vi "srv_loop.vi"(8 "error in (no error)":errorcluster, 9 "Marker Queue":refnum<queue>, 10 "Server queue":refnum<queue>, 11 "Message Queues":T4) -> (0 "error out":errorcluster)   [LabVIEW 2013]
doc: "Message loop for handling messages pertaining to the acquisition of data from the hardware."
uses:
  queues/que_all_message_queues.ctl
  queues/que_message_cluster.ctl
  gui/type_def/general_and_device.ctl
  gui/type_def/general.ctl
  gui/type_def/device.ctl
  srv_state.ctl
  queues/que_enqueue_message_single.vi
  gui/global_var.vi
  <vilib>/Utility/error.llb/Error Cluster From Error Code.vi
  <vilib>/ErrorRing/Error Ring.xnode
panel:
  out "data_format":string
  out "fs":i32
  out "gral_&_device":T1={"general"={"file_ext"="0.0.0.0", "TCP port"=0, "#devices"=0, "log?"=FALSE, "tcp?"=FALSE, "language"="ENG"}, "eeg_device"={"name"="", "hardware"="", "image"="", "path"=path "", "extra"="", "channels"=""}}
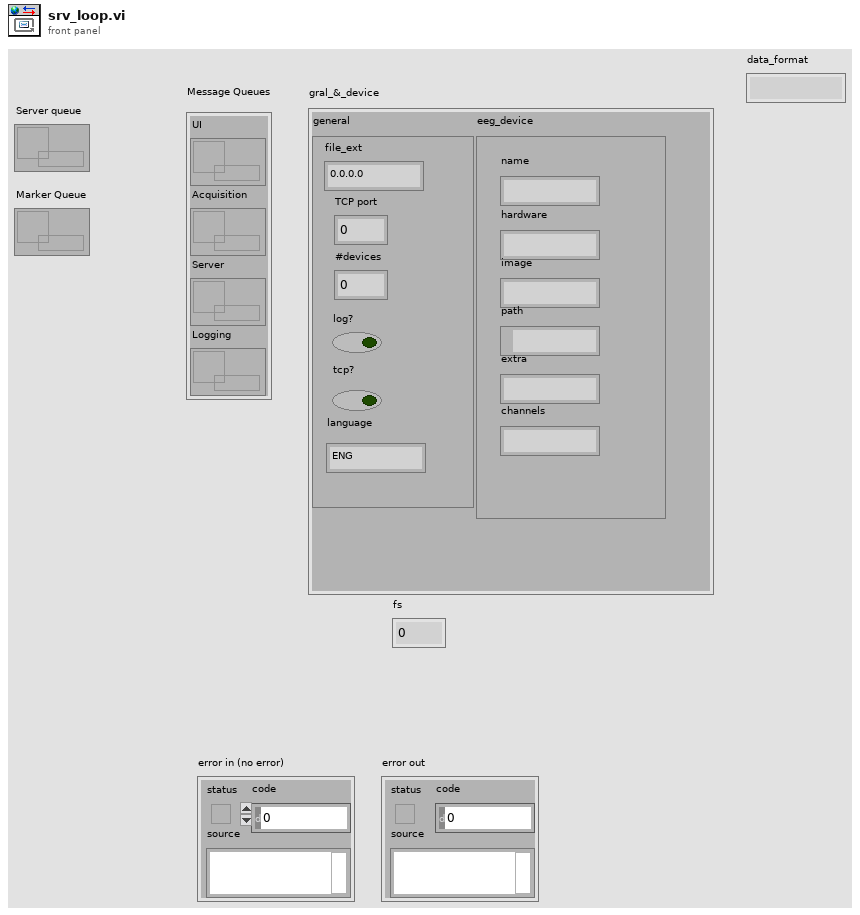
[diagram p1: front panel]
types:
  T1 = typedef "general_and_device.ctl" = cluster{"general":T2, "eeg_device":T3}
  T2 = typedef "general.ctl" = cluster{"file_ext":string, "TCP port":i32, "#devices":i32, "log?":bool, "tcp?":bool, "language":string}
  T3 = typedef "device.ctl" = cluster{"name":string, "hardware":string, "image":string, "path":path, "extra":string, "channels":string}
  T4 = typedef "que_all_message_queues.ctl" = cluster{"UI":refnum<queue>, "Acquisition":refnum<queue>, "Server":refnum<queue>, "Logging":refnum<queue>}
  T5 = typedef "srv_state.ctl" = enum16{"Idle", "Serving"}
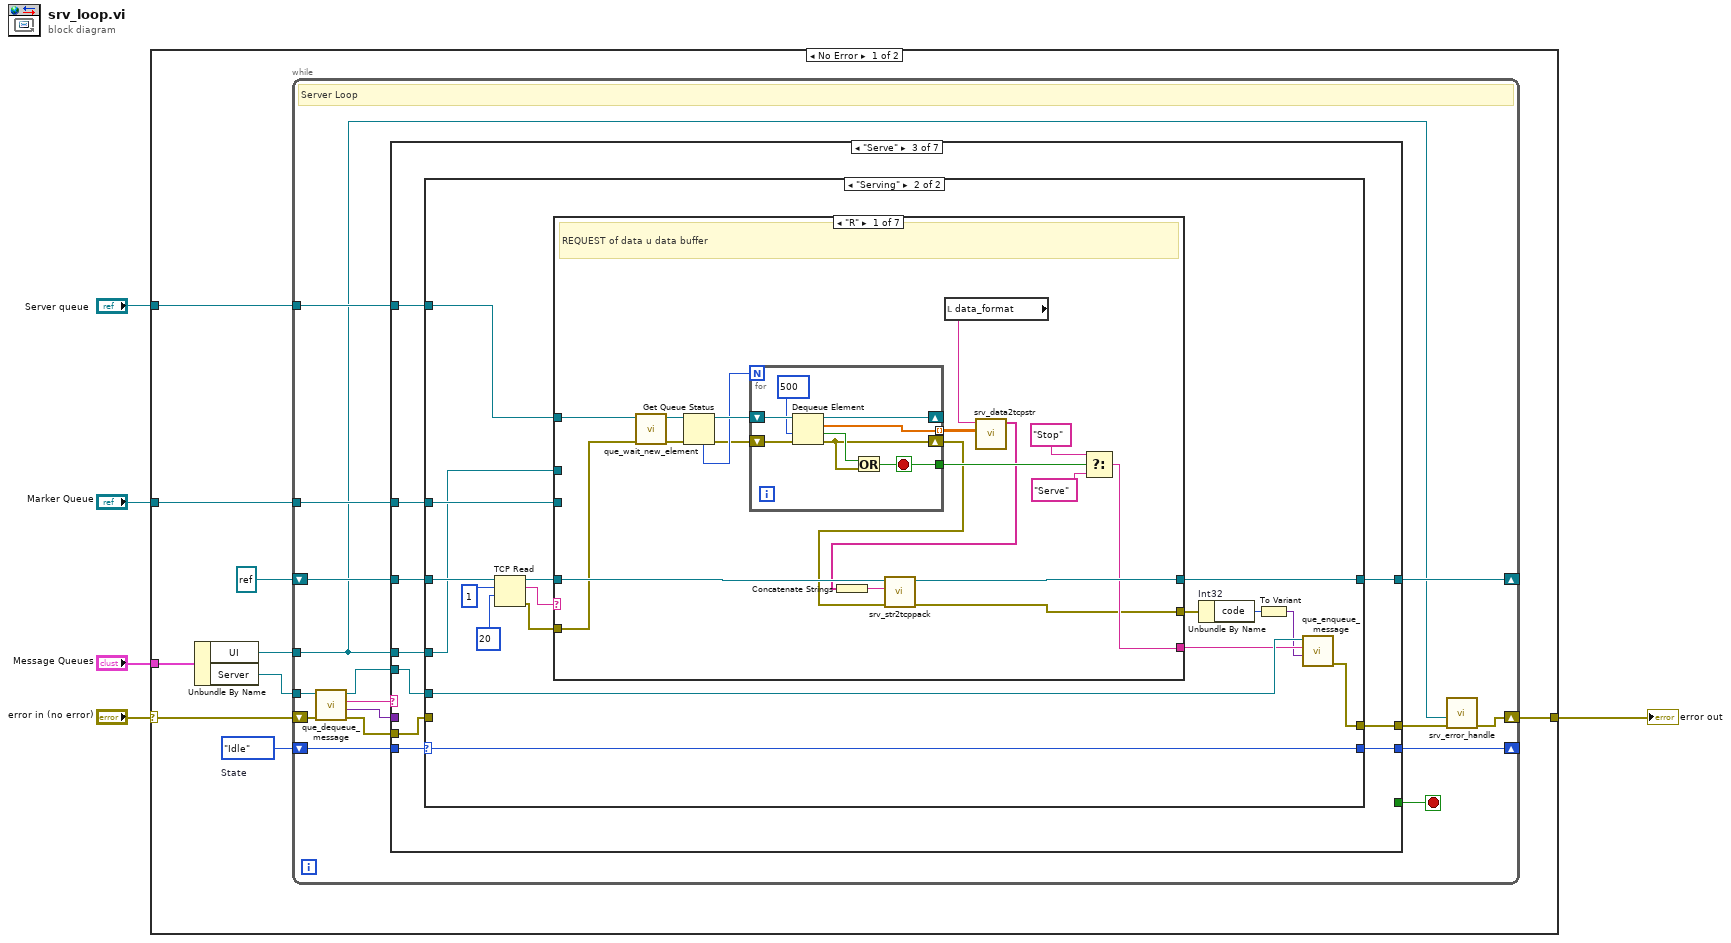
[diagram p0: block diagram]
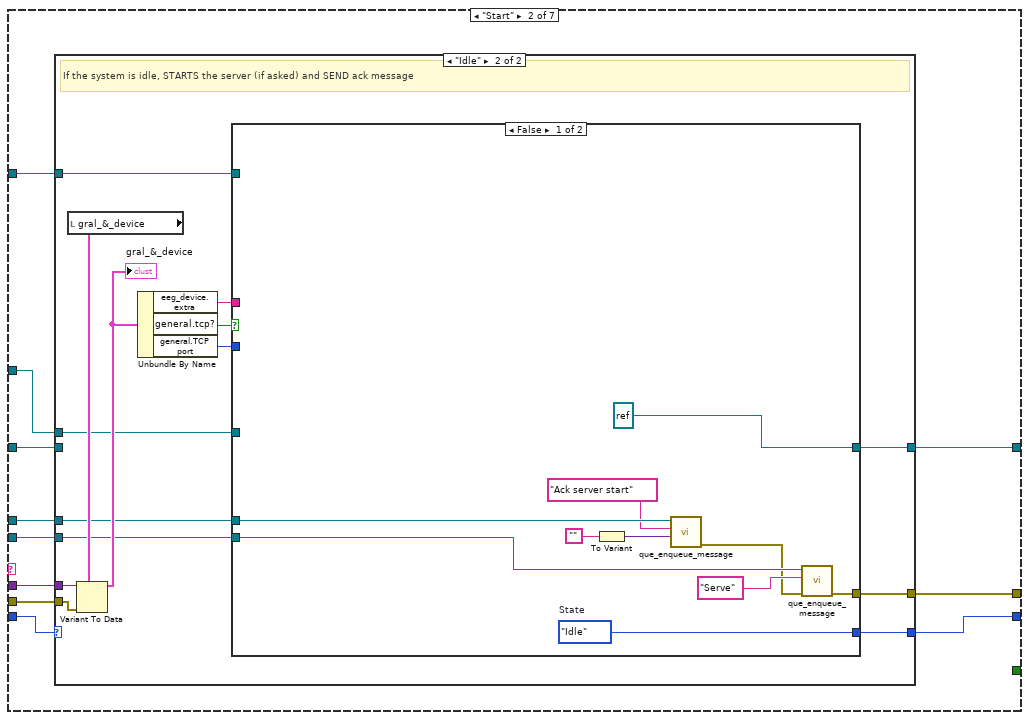
[diagram p3: hidden frame]
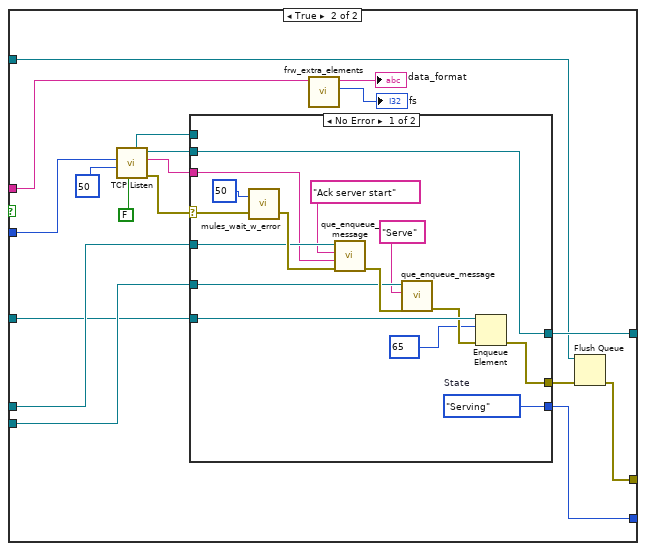
[diagram p5: hidden frame]
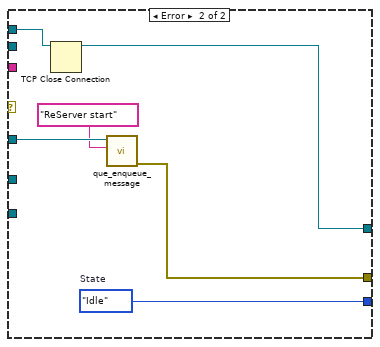
[diagram p6: hidden frame]
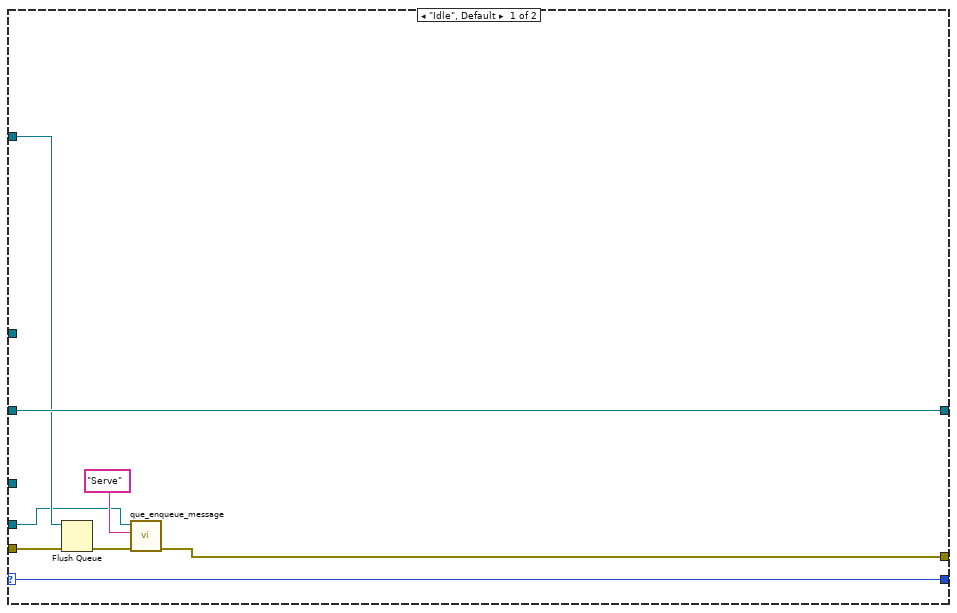
[diagram p7: hidden frame]
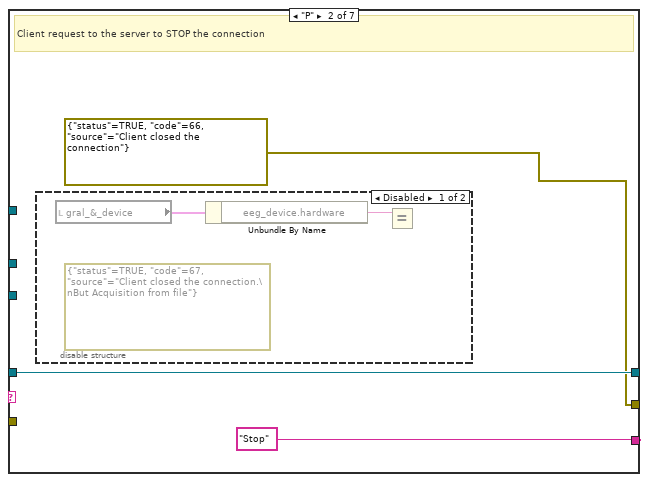
[diagram p8: hidden frame]
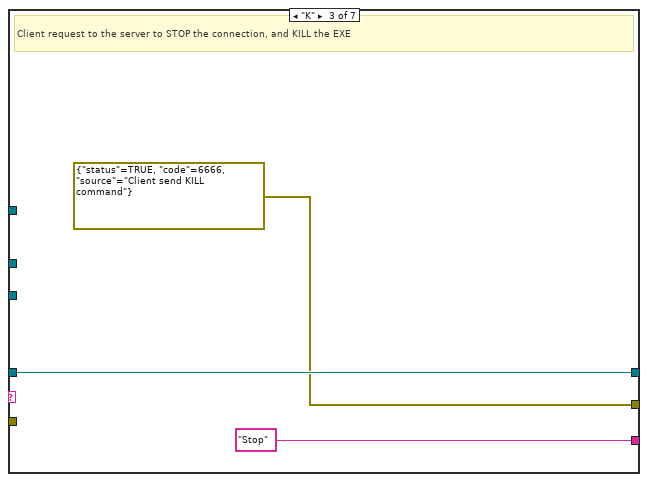
[diagram p10: hidden frame]
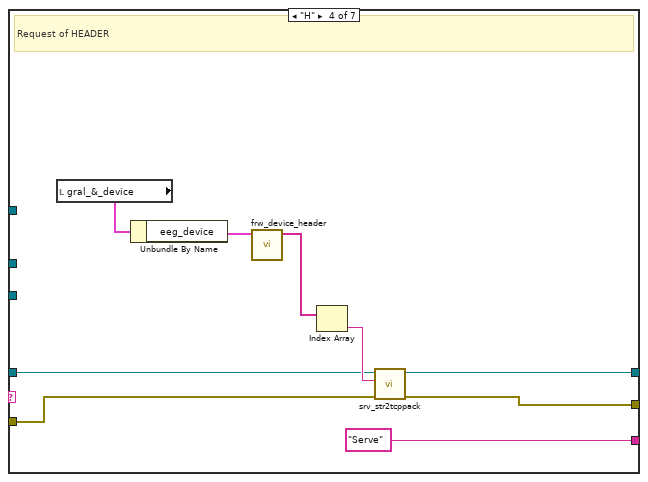
[diagram p11: hidden frame]
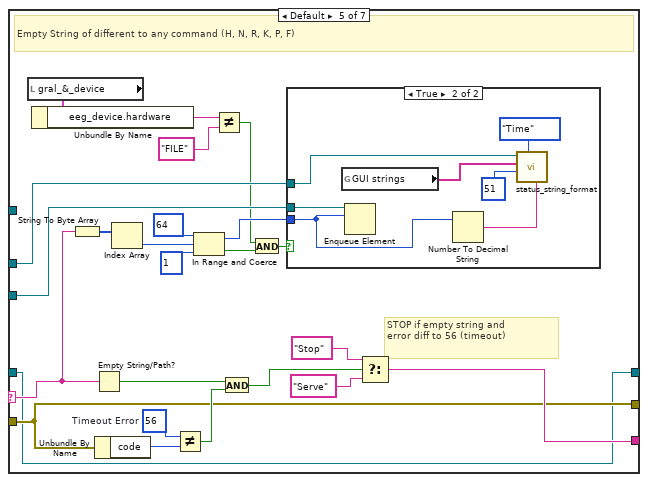
[diagram p12: hidden frame]
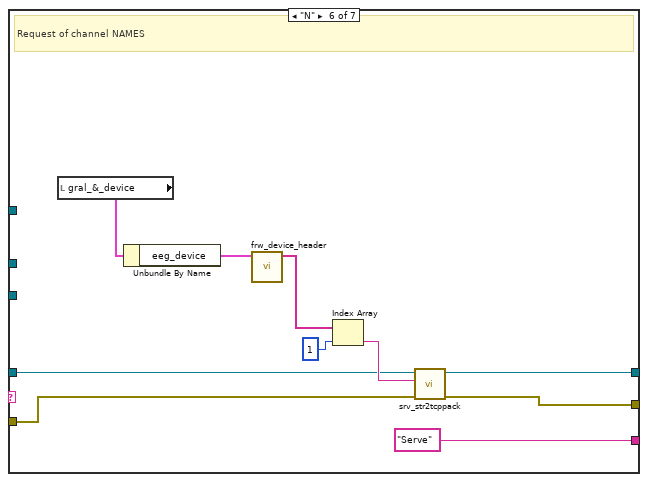
[diagram p14: hidden frame]
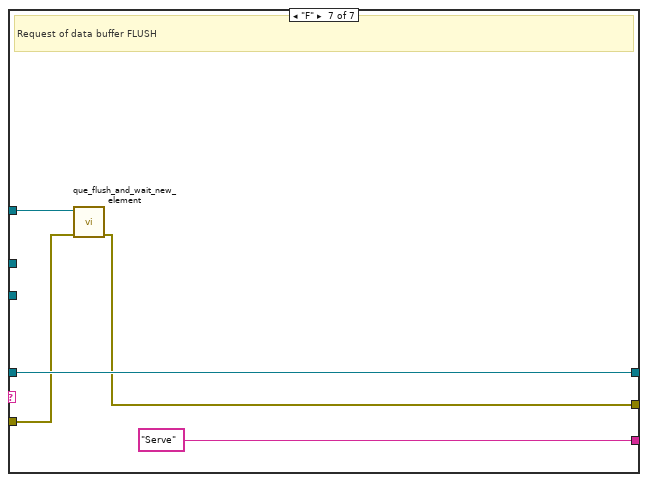
[diagram p15: hidden frame]
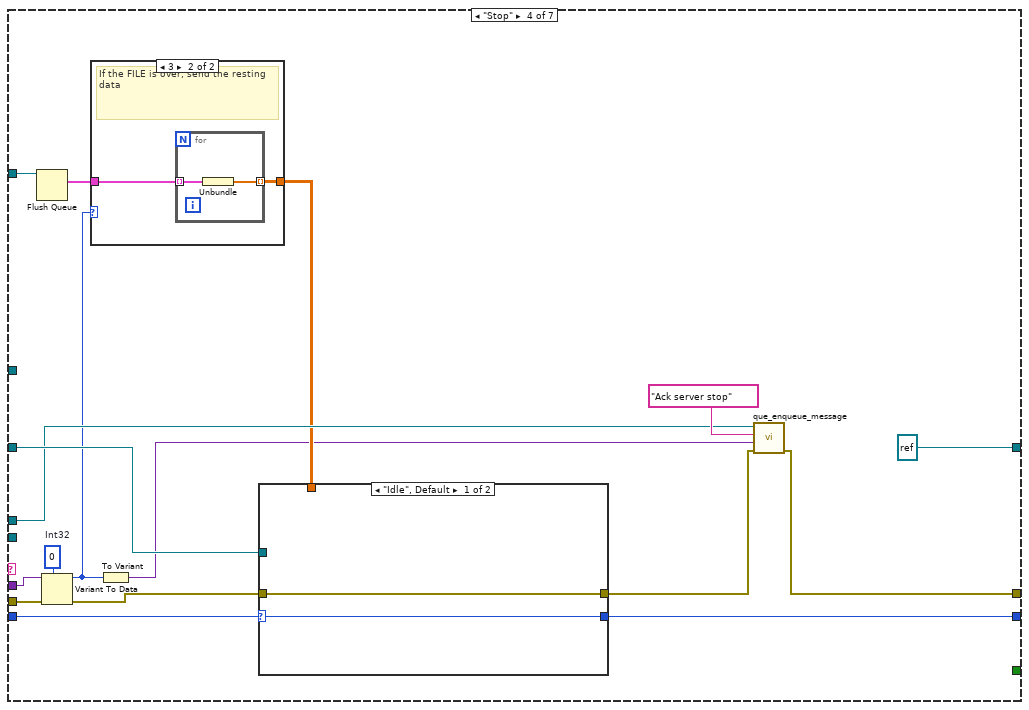
[diagram p16: hidden frame]
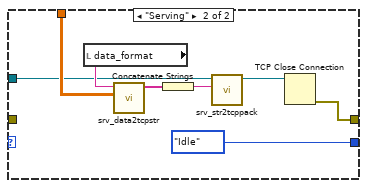
[diagram p18: hidden frame]
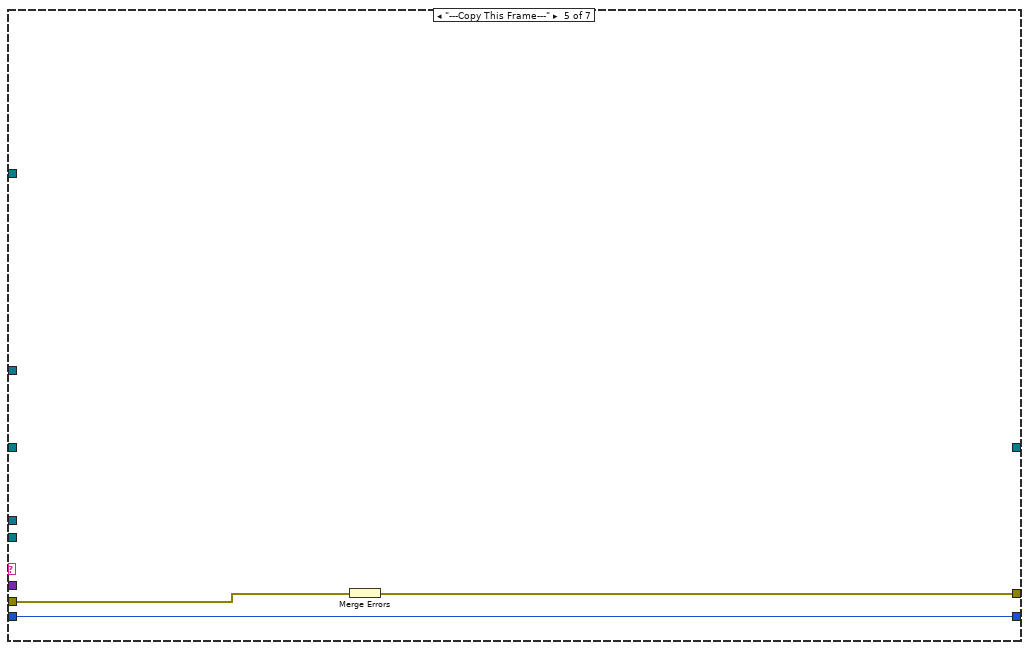
[diagram p19: hidden frame]
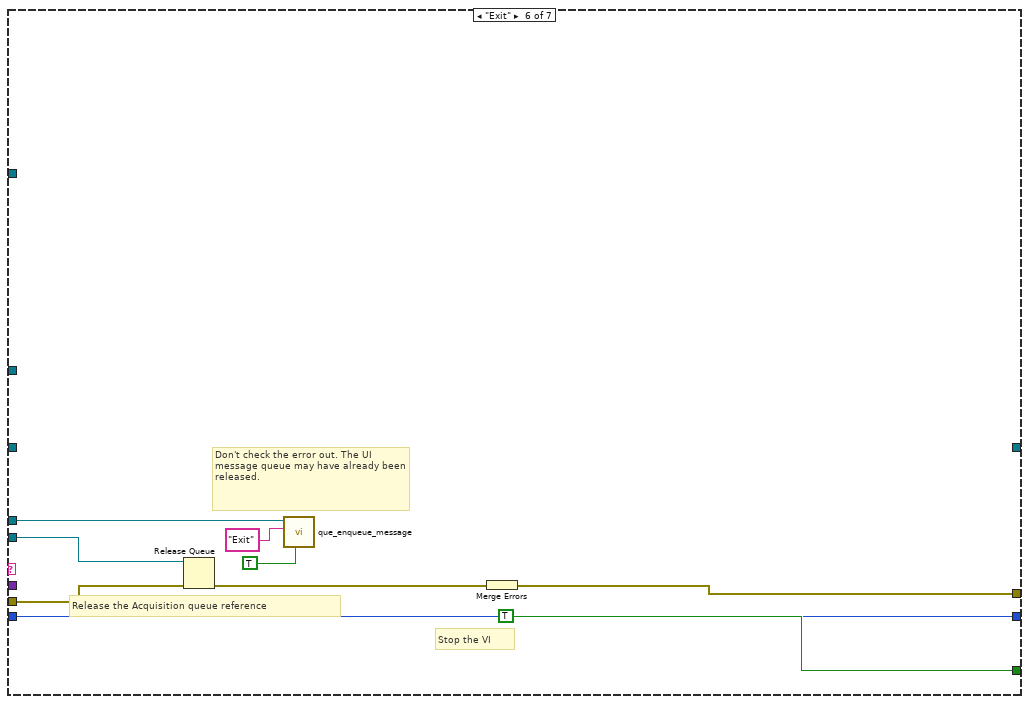
[diagram p20: hidden frame]
diagram:
  n1 = case shown="No Error" "error in (no error)" {
    selector: "error in (no error)" -> [w11 w290]
    tunnel: "Message Queues" -> [w14 _]
    tunnel: [w12 w290] -> w4
    tunnel: "Server queue" -> [w8 _]
    tunnel: "Marker Queue" -> [w6 _]
    frame No Error {
      w9 = srv_state."Idle"  # State
      n2 = Unbundle By Name(w14) -> ("UI"=w10:refnum<queue>, "Server"=w13:refnum<queue>)
      n3 = while {
        tunnel: w13 -> [w26]
        shift-right: [w23] -> w12
        shift-left: w11 -> [w29]
        tunnel: w10 -> [w16]
        shift-right: [w24] -> _
        shift-left: w9 -> [w25]
        tunnel: w8 -> [w20]
        shift-right: [w19] -> _
        shift-left: refnum<k5> refnum ("connection ID out") -> [w18]
        tunnel: w6 -> [w17]
        stop <- w30 stop-if-true
        # "Server Loop"
        n4 = call "que_dequeue_message.vi"("error in (no error)"=w29, "Message Queue"=w26) -> ("error out"=w28:errorcluster, "Message Data"=w27:variant, "Message"=w15:string, "dup Message Queue"=w21:refnum<queue>)  [unwired: 6 in]
        n5 = case "Message Cases" shown="\"Serve\"" w15 {
          selector: w15 -> [_ _ _ _ _ _ w280]
          tunnel: w21 -> [_ w43 w119 _ _ w271 _]
          tunnel: w28 -> [w31 w35 w118 w244 w269 w275 _]
          tunnel: [w31 w44 w120 w237 w268 w277 w281] -> w22
          tunnel: [_ _ _ _ _ TRUE _] -> w30
          tunnel: w27 -> [_ w40 _ w243 _ _ _]
          tunnel: w16 -> [_ w36 w112 w246 _ w276 _]
          tunnel: w25 -> [w33 w41 w116 w252 w267 w270 w282]
          tunnel: [w33 w42 w117 w249 w267 w270 w282] -> w24
          tunnel: w20 -> [_ w39 w115 w239 _ _ _]
          tunnel: [w32 w38 w113 refnum<k5> refnum ("connection ID out") _ _ w279] -> w19
          tunnel: w18 -> [w32 w37 w114 w251 _ _ w279]
          tunnel: w17 -> [_ w34 w111 _ _ _ _]
          frame "Initialize" {
            # "Initialize  - Initialize is currently a no-op.  The EEG initialization is done with the 'start' message."
          }
          frame "Start" {
            n6 = case shown="\"Idle\"" w41 {
              selector: w41 -> [w45 _]
              tunnel: [w46 w51] -> w44
              tunnel: w35 -> [w46 w60]
              tunnel: w43 -> [_ w53]
              tunnel: [w45 w54] -> w42
              tunnel: w40 -> [_ w61]
              tunnel: w39 -> [_ w48]
              tunnel: [w47 w52] -> w38
              tunnel: w37 -> [w47 _]
              tunnel: w36 -> [_ w55]
              tunnel: w34 -> [_ w49]
              frame "Serving" {
                # "The system is already acquiring. Ignore the \"Start\" message."
              }
              frame "Idle" {
                # "If the system is idle, STARTS the server (if asked) and SEND ack message"
                n7 = local read "gral_&_device"() -> (w58:T1)
                n8 = Variant To Data(error in=w60, type=w58, Variant=w61) -> (data=w59:T1)  [unwired: 1 out]
                "gral_&_device" <- w59
                n9 = Unbundle By Name(w59) -> ("eeg_device.extra"=w50:string, "general.tcp?"=w57:bool, "general.TCP port"=w56:i32)
                n10 = case shown="False" w57 {
                  tunnel: w56 -> [_ w88]
                  tunnel: w55 -> [w67 w87]
                  tunnel: [w71 w86] -> w54
                  tunnel: w53 -> [w68 w85]
                  tunnel: [refnum<k5> refnum ("connection ID out") w77] -> w52
                  tunnel: [w64 w75] -> w51
                  tunnel: w50 -> [_ w80]
                  tunnel: w49 -> [_ w78]
                  tunnel: w48 -> [_ w74]
                  frame False {
                    w71 = srv_state."Idle"  # State
                    n11 = To Variant(anything="") -> (Variant=w62:variant)
                    n12 = call-poly "que_enqueue_message.vi"("Message Data"=w62, "Message"="Ack server start", "Message Queue"=w67) -> ("error out"=w65:errorcluster)  [unwired: 7 in, 1 out]
                    n13 = call-poly "que_enqueue_message.vi"("error in (no error)"=w65, "Message"="Serve", "Message Queue"=w68) -> ("error out"=w64:errorcluster)  [unwired: 7 in, 1 out]
                  }
                  frame True {
                    n14 = call <vilib>:"TCP Listen.vi"("resolve remote address (T)"=FALSE, "timeout ms (wait forever: -1)"=50, "port"=w88) -> ("error out"=w82:errorcluster, "remote address"=w83:string, "connection ID"=w72:refnum<k5>, "listener ID"=w73:refnum<k5>)  [unwired: 4 in, 1 out]
                    n15 = case shown="No Error" w82 {
                      selector: w82 -> [w95 _]
                      tunnel: w87 -> [w102 w109]
                      tunnel: [w100 w110] -> w86
                      tunnel: w85 -> [w98 _]
                      tunnel: [w92 w107] -> w76
                      tunnel: w83 -> [w96 _]
                      tunnel: w78 -> [w94 _]
                      tunnel: [w90 w106] -> w77
                      tunnel: w73 -> [_ w105]
                      tunnel: w72 -> [w90 _]
                      frame No Error {
                        w100 = srv_state."Serving"  # State
                        n16 = call "mules_wait_w_error.vi"("error in (no error)"=w95, "milliseconds to wait"=u32 50) -> ("error out"=w103:errorcluster)  [unwired: 1 in]
                        n17 = call-poly "que_enqueue_message.vi"("error in (no error)"=w103, "Message Data"=w96, "Message"="Ack server start", "Message Queue"=w102) -> ("error out"=w99:errorcluster)  [unwired: 6 in, 1 out]
                        n18 = call-poly "que_enqueue_message.vi"("error in (no error)"=w99, "Message"="Serve", "Message Queue"=w98) -> ("error out"=w93:errorcluster)  [unwired: 7 in, 1 out]
                        n19 = Enqueue Element(queue=w94, element=u8 65 ("y"), error in (no error)=w93) -> (error out=w92:errorcluster)  [unwired: 1 in, 2 out]
                      }
                      frame Error {
                        w110 = srv_state."Idle"  # State
                        n20 = TCP Close Connection(connection ID=w105) -> (connection ID out=w106:refnum<k5>)  [unwired: 2 in, 1 out]
                        n21 = call-poly "que_enqueue_message.vi"("Message"="ReServer start", "Message Queue"=w109) -> ("error out"=w107:errorcluster)  [unwired: 8 in, 1 out]
                      }
                    }
                    n22 = call "frw_extra_elements.vi"("string"=w80) -> ("fs"=→"fs":i32, "data_format"=→"data_format":string)  [unwired: 6 in, 3 out]
                    n23 = Flush Queue(queue=w74, error in (no error)=w76) -> (error out=w75:errorcluster)  [unwired: 2 out]
                  }
                }
              }
            }
          }
          frame "Serve" {
            # "Log - Write the data from the eeg  hardware. Since this is a continuous log , this message will always message itself to run again."
            n24 = case shown="\"Serving\"" w116 {
              selector: w116 -> [w128 w145]
              tunnel: [w123 w144] -> w120
              tunnel: w119 -> [w122 w143]
              tunnel: w118 -> [w125 _]
              tunnel: [w128 w145] -> w117
              tunnel: w115 -> [w126 w137]
              tunnel: w114 -> [w127 w141]
              tunnel: [w127 w138] -> w113
              tunnel: w112 -> [_ w129]
              tunnel: w111 -> [_ w132]
              frame "Idle", Default {
                # "Ignore \"Acquire\" messages when the acquisition is idle."
                n25 = Flush Queue(queue=w126, error in (no error)=w125) -> (error out=w121:errorcluster)  [unwired: 2 out]
                n26 = call-poly "que_enqueue_message.vi"("error in (no error)"=w121, "Message"="Serve", "Message Queue"=w122) -> ("error out"=w123:errorcluster)  [unwired: 7 in, 1 out]
              }
              frame "Serving" {
                # "Acquire more data while in the \"Acquiring\" state."
                n27 = TCP Read(connection ID=w141, bytes to read=1, 9:20 ("timeout ms (25000)")) -> (connection ID out=w139:refnum<k5>, data out=w140:string, error out=w134:errorcluster)  [unwired: 2 in]
                n28 = case shown="\"R\"" w140 {
                  selector: w140 -> [_ _ _ _ w206 _ _]
                  tunnel: w139 -> [w161 w174 w180 w185 w192 w226 w235]
                  tunnel: [w162 w174 w180 w184 w192 w225 w235] -> w138
                  tunnel: w137 -> [w147 _ _ _ _ _ w233]
                  tunnel: [w160 "Stop" "Stop" "Serve" w201 "Serve" "Serve"] -> w136
                  tunnel: w134 -> [w146 _ _ w181 w200 w222 w232]
                  tunnel: [w150 errorcluster {"status"=TRUE, "code"=66, "source"="Client closed the connection"} ("error out 2") errorcluster {"status"=TRUE, "code"=6666, "source"="Client send KILL command"} ("error out 2") w182 w200 w221 w231] -> w133
                  tunnel: w132 -> [_ _ _ _ w209 _ _]
                  tunnel: w129 -> [_ _ _ _ w207 _ _]
                  frame "R" {
                    # "REQUEST of data u data buffer"
                    n29 = call "que_wait_new_element.vi"("error in (no error)"=w146, "queue in"=w147) -> ("error out"=w149:errorcluster, "queue out"=w148:refnum<queue>)  [unwired: 8 in]
                    n30 = Get Queue Status(queue=w148, error in (no error)=w149) -> (queue out=w154:refnum<queue>, error out=w151:errorcluster, # elements in queue=w153:i32)  [unwired: 1 in, 5 out]
                    n31 = for {
                      N: w153 -> [_]
                      shift-right: [w171] -> _
                      shift-left: w154 -> [w172]
                      tunnel: [w170] -> w164 mode=indexing
                      tunnel: [w167] -> w157
                      shift-right: [w165] -> w152
                      shift-left: w151 -> [w168]
                      stop <- w167 stop-if-true
                      n32 = Dequeue Element(queue=w172, timeout in ms (-1)=500, error in (no error)=w168) -> (queue out=w171:refnum<queue>, element=w170:dbl[], timed out?=w166:bool, error out=w165:errorcluster)
                      n33 = Or(x=w166, y=w165) -> (x .or. y?=w167:bool)
                    }
                    n34 = local read "data_format"() -> (w163:string)
                    n35 = call "srv_data2tcpstr.vi"("values"=w164, "tags"=w163) -> ("string array"=w155:string[])  [unwired: 9 in]
                    n36 = Concatenate Strings(w155) -> (w156:string)
                    n37 = call "srv_str2tcppack.vi"("error in"=w152, "string  in"=w156, "connection ID"=w161) -> ("error out"=w150:errorcluster, "connection ID out"=w162:refnum<k5>)  [unwired: 7 in]
                    n38 = Select(t="Stop", s=w157, f="Serve") -> (s? t:f=w160:string)
                  }
                  frame "P" {
                    # "Client request to the server to STOP the connection"
                    n39 = disable-structure shown="Disabled" {
                      frame Disabled {
                        (unwired) errorcluster {"status"=TRUE, "code"=67, "source"="Client closed the connection.\nBut Acquisition from file"} ("error out 2")
                        n40 = local read "gral_&_device"() -> (w177:T1)
                        n41 = Unbundle By Name(w177) -> ("eeg_device.hardware"=w176:string)
                        n42 = Equal?(x=w176) -> ()  [unwired: 1 in, 1 out]
                      }
                      frame Enabled {
                      }
                    }
                  }
                  frame "K" {
                    # "Client request to the server to STOP the connection, and KILL the EXE"
                  }
                  frame "H" {
                    # "Request of HEADER"
                    n43 = local read "gral_&_device"() -> (w189:T1)
                    n44 = Unbundle By Name(w189) -> ("eeg_device"=w188:T3)
                    n45 = call "frw_device_header.vi"("eeg_device"=w188) -> ("header array"=w187:string[])  [unwired: 10 in]
                    n46 = Index Array(array=w187) -> (element=w186:string)  [unwired: 1 in]
                    n47 = call "srv_str2tcppack.vi"("error in"=w181, "string  in"=w186, "connection ID"=w185) -> ("error out"=w182:errorcluster, "connection ID out"=w184:refnum<k5>)  [unwired: 7 in]
                  }
                  frame Default {
                    w204 = 56  # Timeout Error
                    # "STOP if empty string and \nerror diff to 56 (timeout)"
                    # "Empty String of different to any command (H, N, R, K, P, F)"
                    n48 = local read "gral_&_device"() -> (w196:T1)
                    n49 = Unbundle By Name(w196) -> ("eeg_device.hardware"=w195:string)
                    n50 = String To Byte Array(string=w206) -> (unsigned byte array=w213:u8[])
                    n51 = Empty String/Path?(string/path=w206) -> (empty?=w199:bool)
                    n52 = Unbundle By Name ("Int32")(w200) -> ("code"=w205:i32)
                    n53 = Index Array(array=w213) -> (element=w210:u8)  [unwired: 1 in]
                    n54 = Not Equal?(x=w204, y=w205) -> (x != y?=w202:bool)
                    n55 = In Range and Coerce(upper limit=u8 64 ("Char"), x=w210, lower limit=u8 1 ("Char")) -> (coerced(x)=w208:u8, In Range?=w190:bool)
                    n56 = Not Equal?(x=w195, y="FILE") -> (x != y?=w191:bool)
                    n57 = And(x=w199, y=w202) -> (x .and. y?=w203:bool)
                    n58 = And(x=w191, y=w190) -> (x .and. y?=w193:bool)
                    n59 = case shown="True" w193 {
                      tunnel: w209 -> [_ w220]
                      tunnel: w208 -> [_ w214]
                      tunnel: w207 -> [_ w216]
                      frame False {
                      }
                      frame True {
                        n60 = global read "global_var.vi" "GUI strings"() -> (w218:string[])
                        n61 = Enqueue Element(queue=w220, element=w214) -> ()  [unwired: 2 in, 3 out]
                        n62 = Number To Decimal String(number=w214) -> (decimal integer string=w215:string)  [unwired: 1 in]
                        n63 = call "status_string_format.vi"("marker"=w215, "color"=enum16{"Black", "Blue", "Red", "Time"}."Time", "index"=51, "gui_strings"=w218, "Message Queue"=w216) -> ()  [unwired: 5 in, 2 out]
                      }
                    }
                    n64 = Select(t="Stop", s=w203, f="Serve") -> (s? t:f=w201:string)
                  }
                  frame "N" {
                    # "Request of channel NAMES"
                    n65 = local read "gral_&_device"() -> (w230:T1)
                    n66 = Unbundle By Name(w230) -> ("eeg_device"=w229:T3)
                    n67 = call "frw_device_header.vi"("eeg_device"=w229) -> ("header array"=w228:string[])  [unwired: 10 in]
                    n68 = Index Array(array=w228, index=1) -> (element=w227:string)
                    n69 = call "srv_str2tcppack.vi"("error in"=w222, "string  in"=w227, "connection ID"=w226) -> ("error out"=w221:errorcluster, "connection ID out"=w225:refnum<k5>)  [unwired: 7 in]
                  }
                  frame "F" {
                    # "Request of data buffer FLUSH"
                    n70 = call "que_flush_and_wait_new_element.vi"("error in (no error)"=w232, "queue in"=w233) -> ("error out"=w231:errorcluster)  [unwired: 8 in, 1 out]
                  }
                }
                n71 = Unbundle By Name "Int32"(w133) -> ("code"=w130:i32)
                n72 = To Variant(anything=w130) -> (Variant=w131:variant)
                n73 = call-poly "que_enqueue_message.vi"("Message Data"=w131, "Message"=w136, "Message Queue"=w143) -> ("error out"=w144:errorcluster)  [unwired: 7 in, 1 out]
              }
            }
          }
          frame "Stop" {
            w247 = 0  # Int32
            # "Stop - Stop the Acquisition."
            n74 = Flush Queue(queue=w239) -> (remaining elements=w238:cluster{dbl[]}[])  [unwired: 1 in, 2 out]
            n75 = Variant To Data(error in=w244, type=w247, Variant=w243) -> (data=w240:i32, error out=w241:errorcluster)
            n76 = case shown="3" w240 {
              tunnel: [_ w254] -> w245
              tunnel: w238 -> [_ w253]
              frame 0, Default {
              }
              frame 3 {
                # "If the FILE is over, send the resting data"
                n77 = for {
                  tunnel: w253 -> [w256] mode=indexing
                  tunnel: [w255] -> w254 mode=indexing
                  n78 = Unbundle(w256) -> (w255:dbl[])
                }
              }
            }
            n79 = To Variant(anything=w240) -> (Variant=w242:variant)
            n80 = case shown="\"Idle\", Default" w252 {
              selector: w252 -> [w258 _]
              tunnel: [w257 w259] -> w236
              tunnel: w241 -> [w257 _]
              tunnel: w251 -> [_ w261]
              tunnel: [w258 srv_state."Idle" ("State")] -> w249
              tunnel: w245 -> [_ w262]
              frame "Idle", Default {
              }
              frame "Serving" {
                # "Put in TCP client and save in File if required"
                n81 = local read "data_format"() -> (w265:string)
                n82 = call "srv_data2tcpstr.vi"("values"=w262, "tags"=w265) -> ("string array"=w263:string[])  [unwired: 9 in]
                n83 = Concatenate Strings(w263) -> (w264:string)
                n84 = call "srv_str2tcppack.vi"("string  in"=w264, "connection ID"=w261) -> ("connection ID out"=w260:refnum<k5>)  [unwired: 8 in, 1 out]
                n85 = TCP Close Connection(connection ID=w260) -> (error out=w259:errorcluster)  [unwired: 2 in, 1 out]
              }
            }
            n86 = call-poly "que_enqueue_message.vi"("error in (no error)"=w236, "Message Data"=w242, "Message"="Ack server stop", "Message Queue"=w246) -> ("error out"=w237:errorcluster)  [unwired: 6 in, 1 out]
          }
          frame "---Copy This Frame---" {
            # "Duplicate this frame when creating new messages.  Change this comment in the duplicated frame to describe this message."
            n87 = Merge Errors(w269) -> (w268:errorcluster)
          }
          frame "Exit" {
            # "Don't check the error out. The UI message queue may have already been released."
            # "Release the Acquisition queue reference"
            # "Stop the VI"
            # "Exit - Send the Exit message to the UI Message Handler."
            n88 = Release Queue(queue=w271, error in (no error)=w275) -> (error out=w272:errorcluster)  [unwired: 1 in, 2 out]
            n89 = call-poly "que_enqueue_message.vi"("Priority Message? (F)"=TRUE, "Message"="Exit", "Message Queue"=w276) -> ()  [unwired: 7 in, 2 out]
            n90 = Merge Errors(w272) -> (w277:errorcluster)
          }
          frame Default {
            # "'Default' case only runs if there is a message that isn't defined in any of the other cases.  Output a programming error."
            n91 = xnode "Error Ring"("parameter 0"=w280) -> ("error out"=w281:errorcluster)
          }
        }
        n92 = call "srv_error_handle.vi"("error in (no error)"=w22, "Message Queue"=w16) -> ("dup error in"=w23:errorcluster)  [unwired: 8 in, 1 out]
      }
    }
    frame Error {
    }
  }
  "error out" <- w4
